vi "Init Task.vi"(6 "line grouping":i32(ring) items=["one channel for each line", "one channel for all lines"], 7 "counter":tag, 8 "error in (no error)":errorcluster, 9 "name":string, 10 "physical channels":tag, 11 "DAQmxTaskDOutput_Emulate in":refnum<class "DAQmxTaskDOutput_Emulate.lvclass">) -> (0 "error out":errorcluster, 3 "DAQmxTaskDOutput_Emulate out":refnum<class "DAQmxTaskDOutput_Emulate.lvclass">)   [LabVIEW 2015, in "DAQmxTaskDOutput_Emulate.lvclass"]
uses:
  DAQmxTaskDOutput_Emulate.lvclass
  DAQmxTask.lvclass/DAQmxTask.ctl
  DAQmxTask.lvclass
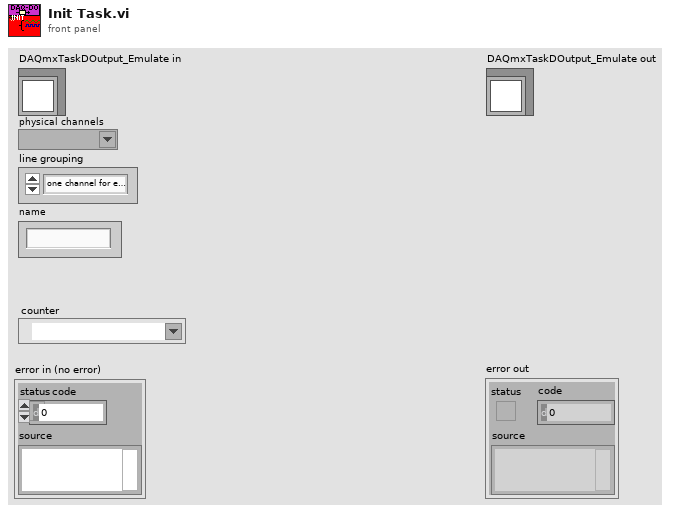
[diagram p1: front panel]
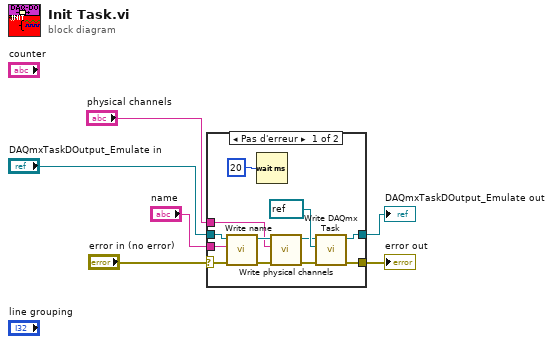
[diagram p0: block diagram]
diagram:
  n1 = case shown="Pas d'erreur" "error in (no error)" {
    selector: "error in (no error)" -> [w13 w19]
    tunnel: "name" -> [w12 _]
    tunnel: "physical channels" -> [w11 _]
    tunnel: [w10 w20] -> w3
    tunnel: [w9 w19] -> w2
    tunnel: "DAQmxTaskDOutput_Emulate in" -> [w8 w20]
    frame No Error {
      n2 = call "Write name.vi"("error in (no error)"=w13, "name"=w12, "DAQmxTask in"=w8) -> ("error out"=w15:errorcluster, "DAQmxTask out"=w16:refnum<class "DAQmxTaskDOutput_Emulate.lvclass">)  [unwired: 7 in]
      n3 = Wait (ms)(milliseconds to wait=u32 20) -> ()  [unwired: 1 out]
      n4 = call "Write physical channels.vi"("error in (no error)"=w15, "physical channels"=w11, "DAQmxTask in"=w16) -> ("error out"=w14:errorcluster, "DAQmxTask out"=w17:refnum<class "DAQmxTaskDOutput_Emulate.lvclass">)  [unwired: 7 in]
      n5 = call "Write DAQmx Task.vi"("error in (no error)"=w14, "DAQmx Task Name"=refnum<k21> refnum, "DAQmxTask in"=w17) -> ("error out"=w9:errorcluster, "DAQmxTask out"=w10:refnum<class "DAQmxTaskDOutput_Emulate.lvclass">)  [unwired: 7 in]
    }
    frame Error {
    }
  }
  "error out" <- w2
  "DAQmxTaskDOutput_Emulate out" <- w3
